vi "添加启动项.vi"(8 "error in (no error)":errorcluster caption="错误输入（无错误）") -> (0 "error out":errorcluster caption="错误输出", 3 "添加成功标记":bool)   [LabVIEW 2016, in "wxpusher.lvlib"]
uses:
  wxpusher.lvlib
  <vilib>/registry/registry.llb/Registry RtKey.ctl
  <vilib>/registry/registry.llb/Write Registry Value Simple STR.vi
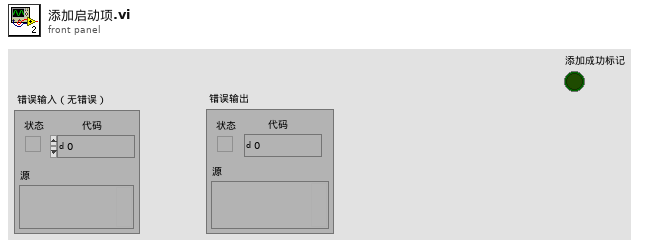
[diagram p1: front panel]
types:
  T1 = typedef "Registry RtKey.ctl" = enum32{"HKEY_CLASSES_ROOT", "HKEY_CURRENT_USER", "HKEY_LOCAL_MACHINE", "HKEY_USERS", "HKEY_PERFORMANCE_DATA", "HKEY_CURRENT_CONFIG", "HKEY_DYN_DATA"}
  T2 = typedef "Registry refnum.ctl" = refnum<k1>
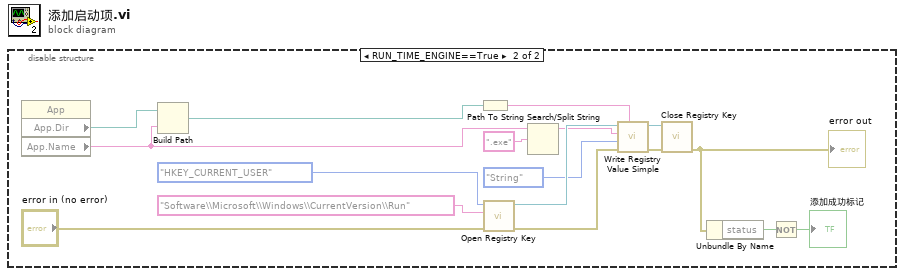
[diagram p0: block diagram]
diagram:
  n1 = disable-structure shown="RUN_TIME_ENGINE==True" {
    frame condition #0 (active) {
    }
    frame condition #1 {
      n2 = property class="App"() -> ("App.Dir"=w4:path, "App.Name"=w3:string)  [unwired: 2 in, 2 out]
      n3 = Build Path(base path=w4, name or relative path=w3) -> (appended path=w5:path)
      n4 = Path To String(path=w5) -> (string=w6:string)
      n5 = call <vilib>:"Open Registry Key.vi"("error in (no error)"="error in (no error)", "subkey"="Software\\Microsoft\\Windows\\CurrentVersion\\Run", "root key (HKEY_LOCAL_MACHINE)"=Registry_RtKey."HKEY_CURRENT_USER") -> ("error out"=w14:errorcluster, "refnum out"=w13:T2)  [unwired: 7 in]
      n6 = Search/Split String(string=w3, search string/char (-)=".exe" ("搜索字符串/字符(-)")) -> (substring before match=w1:string)  [unwired: 1 in, 2 out]
      n7 = call-poly <vilib>:"Write Registry Value Simple.vi"("String/Binary data"=w6, "error in (no error)"=w14, "simple data type"=enum16{"String", "Binary", "DWORD"}."String", "value"=w1, "refnum"=w13) -> ("error out"=w16:errorcluster, "refnum out"=w15:T2)  [unwired: 3 in]
      n8 = call <vilib>:"Close Registry Key.vi"("error in (no error)"=w16, "refnum"=w15) -> ("error out"=w8:errorcluster)  [unwired: 5 in]
      "error out" <- w8
      n9 = Unbundle By Name(w8) -> ("status"=w7:bool)
      n10 = Not(x=w7) -> (.not. x?=→"添加成功标记":bool)
    }
  }
